vi "Photodiode-test.vi"() -> ()   [LabVIEW 2015]
uses:
  PDE_State_Machine_12_12_2016_LabVIEW_15/StateIndicator.ctl
  PDE_State_Machine_12_12_2016_LabVIEW_15/PDEState.ctl
  <vilib>/DAQmx/read.llb/DAQmx Read.vi
  <vilib>/DAQmx/read.llb/DAQmx Read (Analog 1D Wfm NChan NSamp).vi
  <vilib>/DAQmx/create/channels.llb/DAQmx Create Channel (AI-Voltage-Basic).vi
  <vilib>/DAQmx/configure/timing.llb/DAQmx Timing (Sample Clock).vi
  <vilib>/DAQmx/miscellaneous.llb/DAQmx Fill In Error Info.vi
panel:
  in  "error in":errorcluster
  out "Photodiode Values":waveform(dbl)[](graph)
  in  "Test Button":bool
  in  "Go To Idle":bool
  in  "Abort VI":bool
  out "PDE State":T1 items=["Stop VI", "Predet Fire", "Control Button", "Stop", "Connecting", "Firing", "Testing ", "Idle", "Init"]
  in  "Sample Rate (Hz)":dbl(slide)=1.0 min=0.0 max=1000000.0 step=10.0 scale=1.0..1000000.0
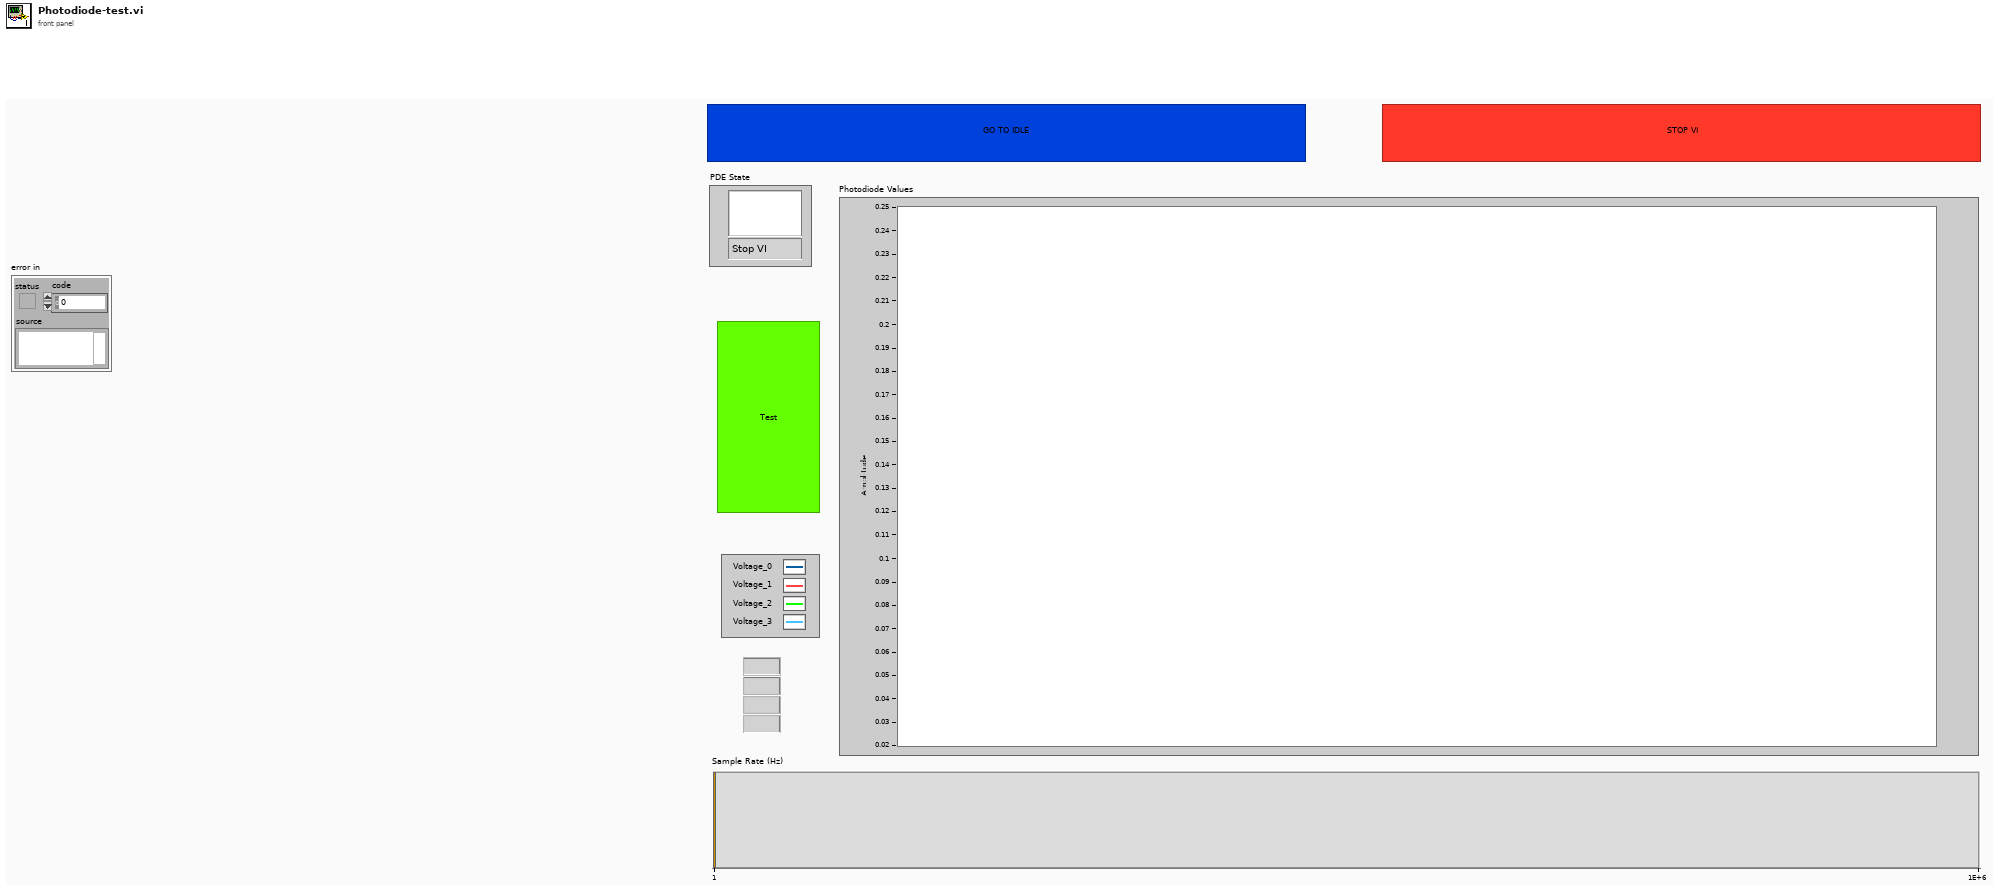
[diagram p1: front panel]
types:
  T1 = typedef "StateIndicator.ctl" = u16
  T2 = typedef "PDEState.ctl" = enum16{"Stop VI", "Predet Fire", "Control Button", "Stop", "Connecting", "Firing ", "Testing ", "Idle", "Init"}
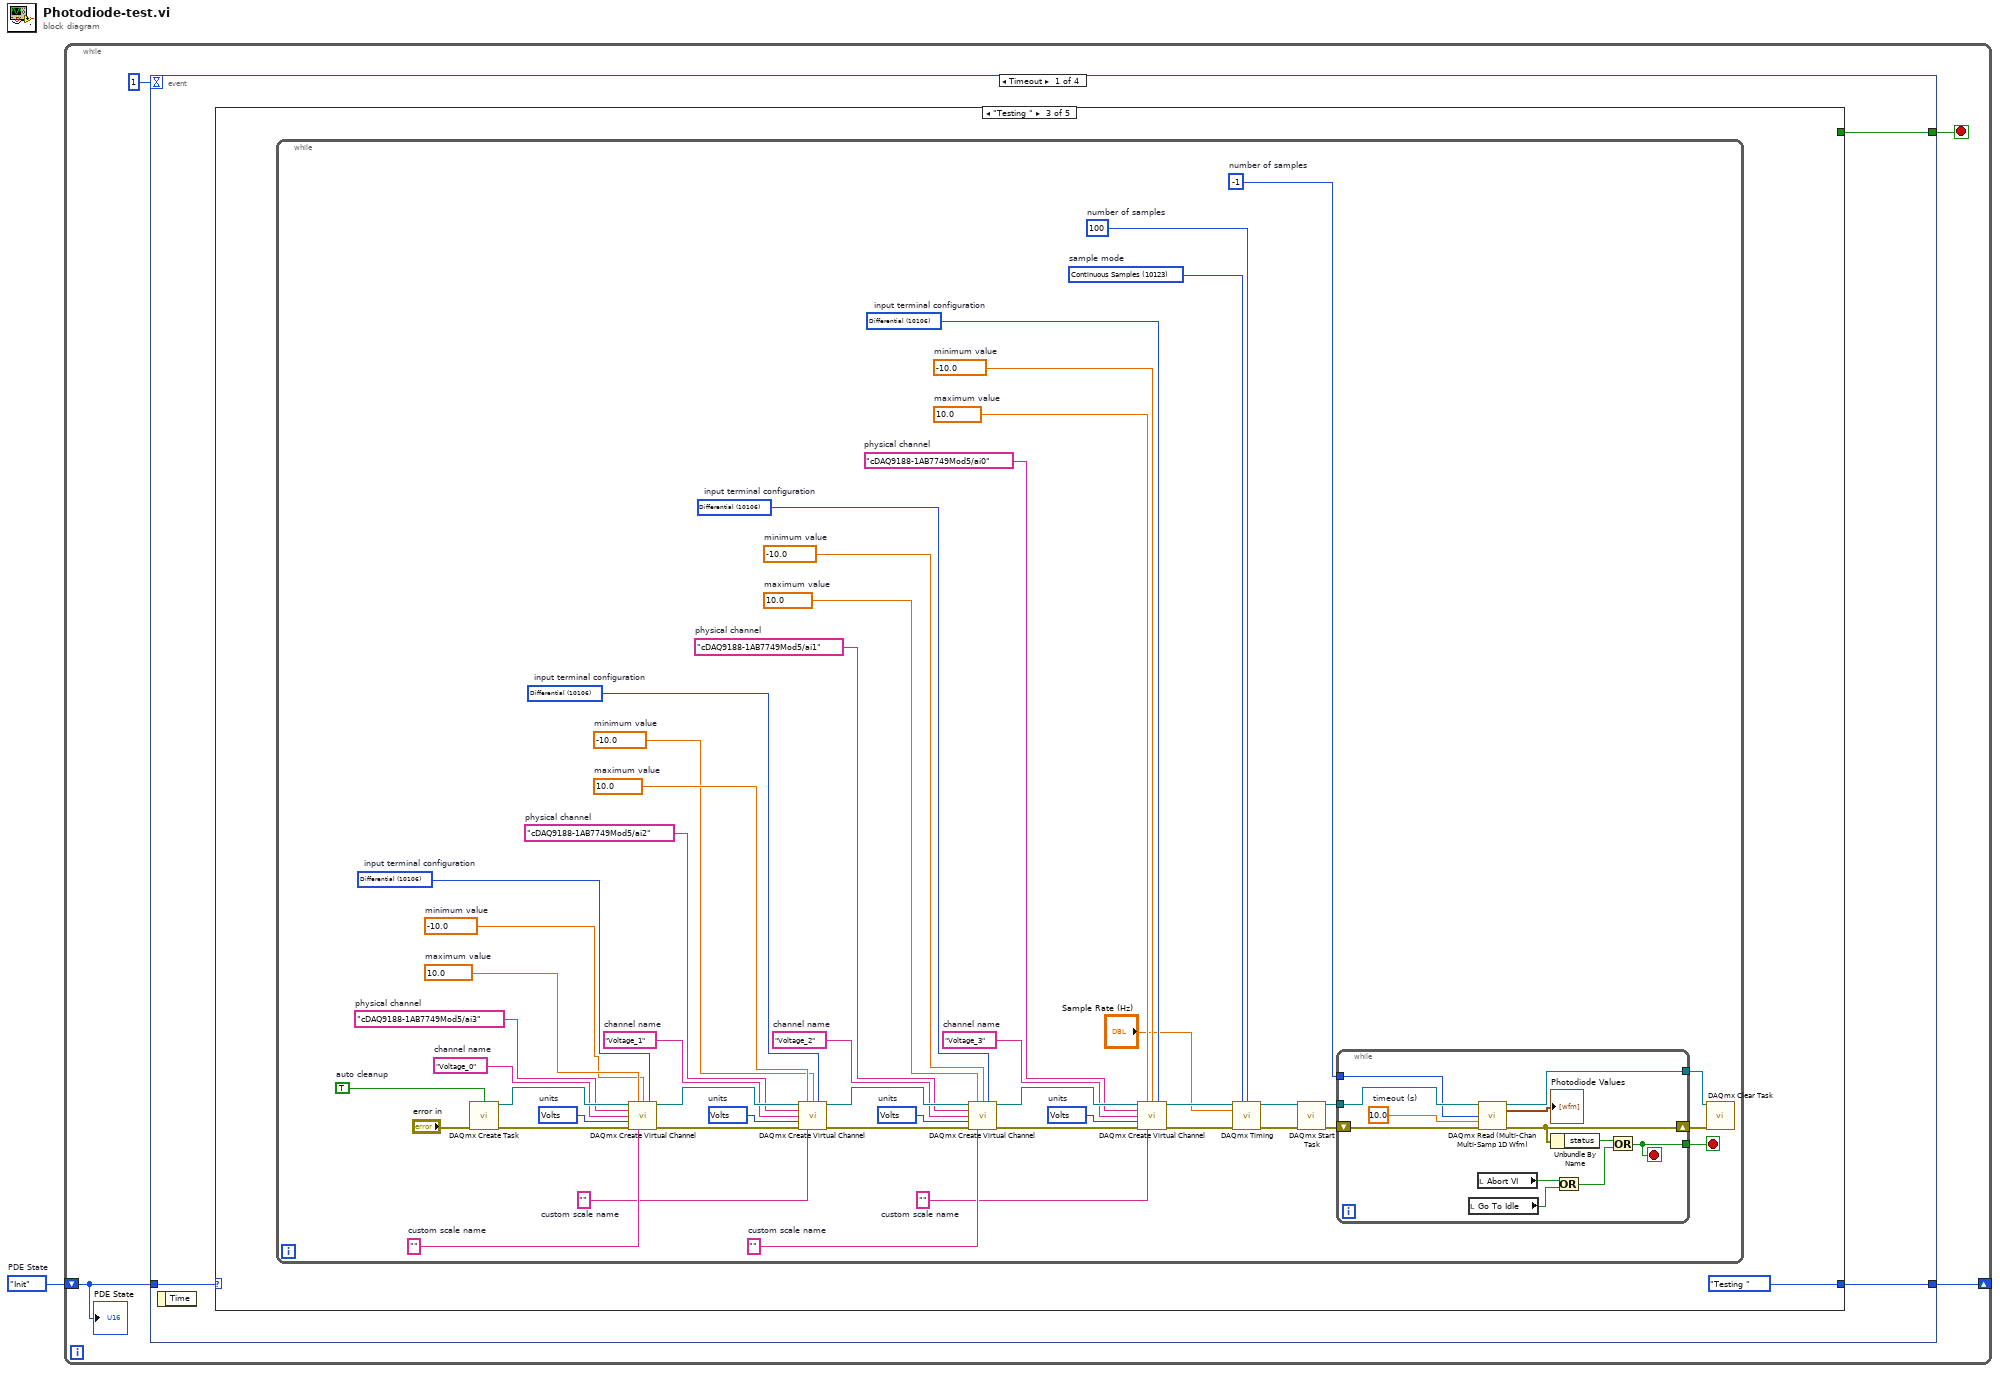
[diagram p0: block diagram]
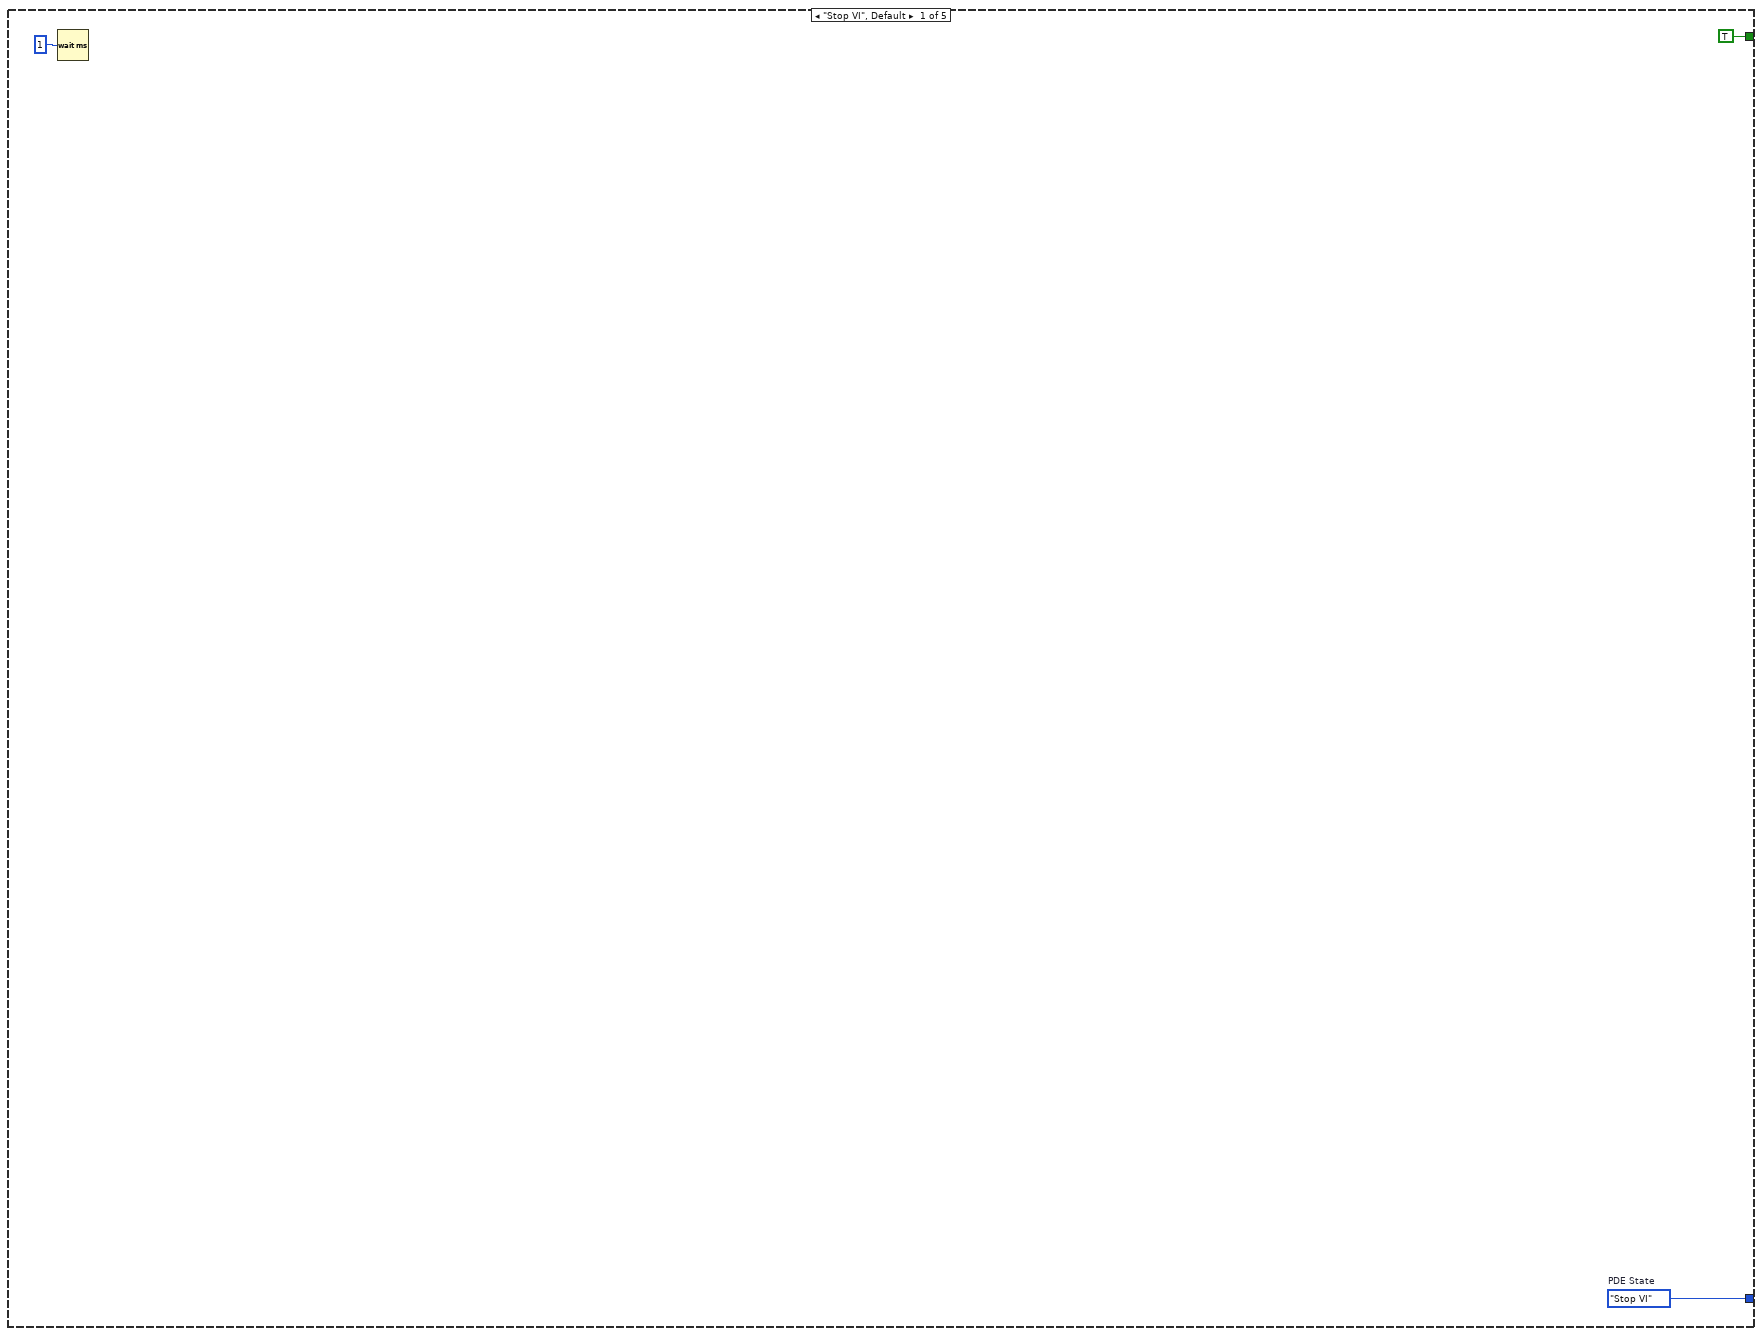
[diagram p2: hidden frame]
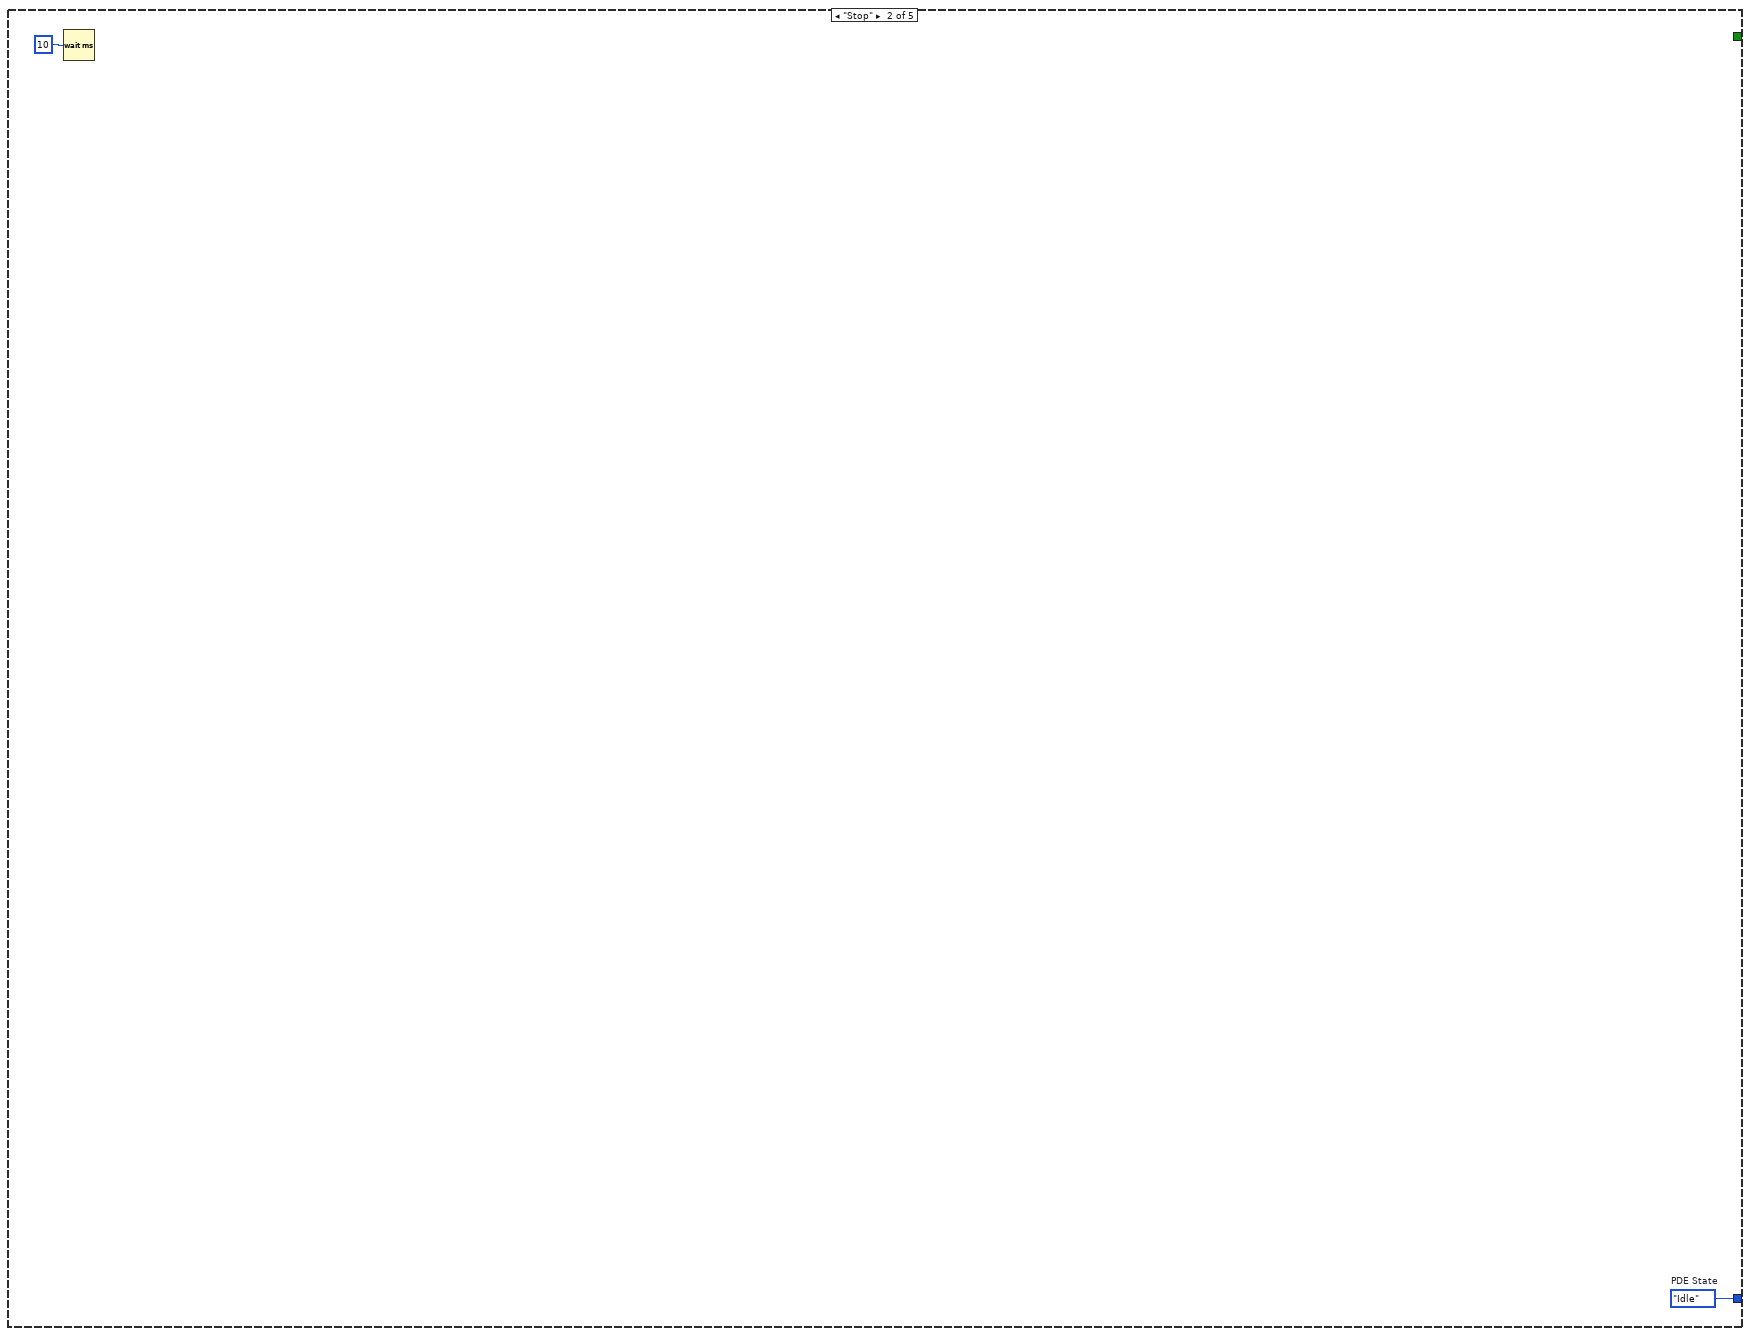
[diagram p3: hidden frame]
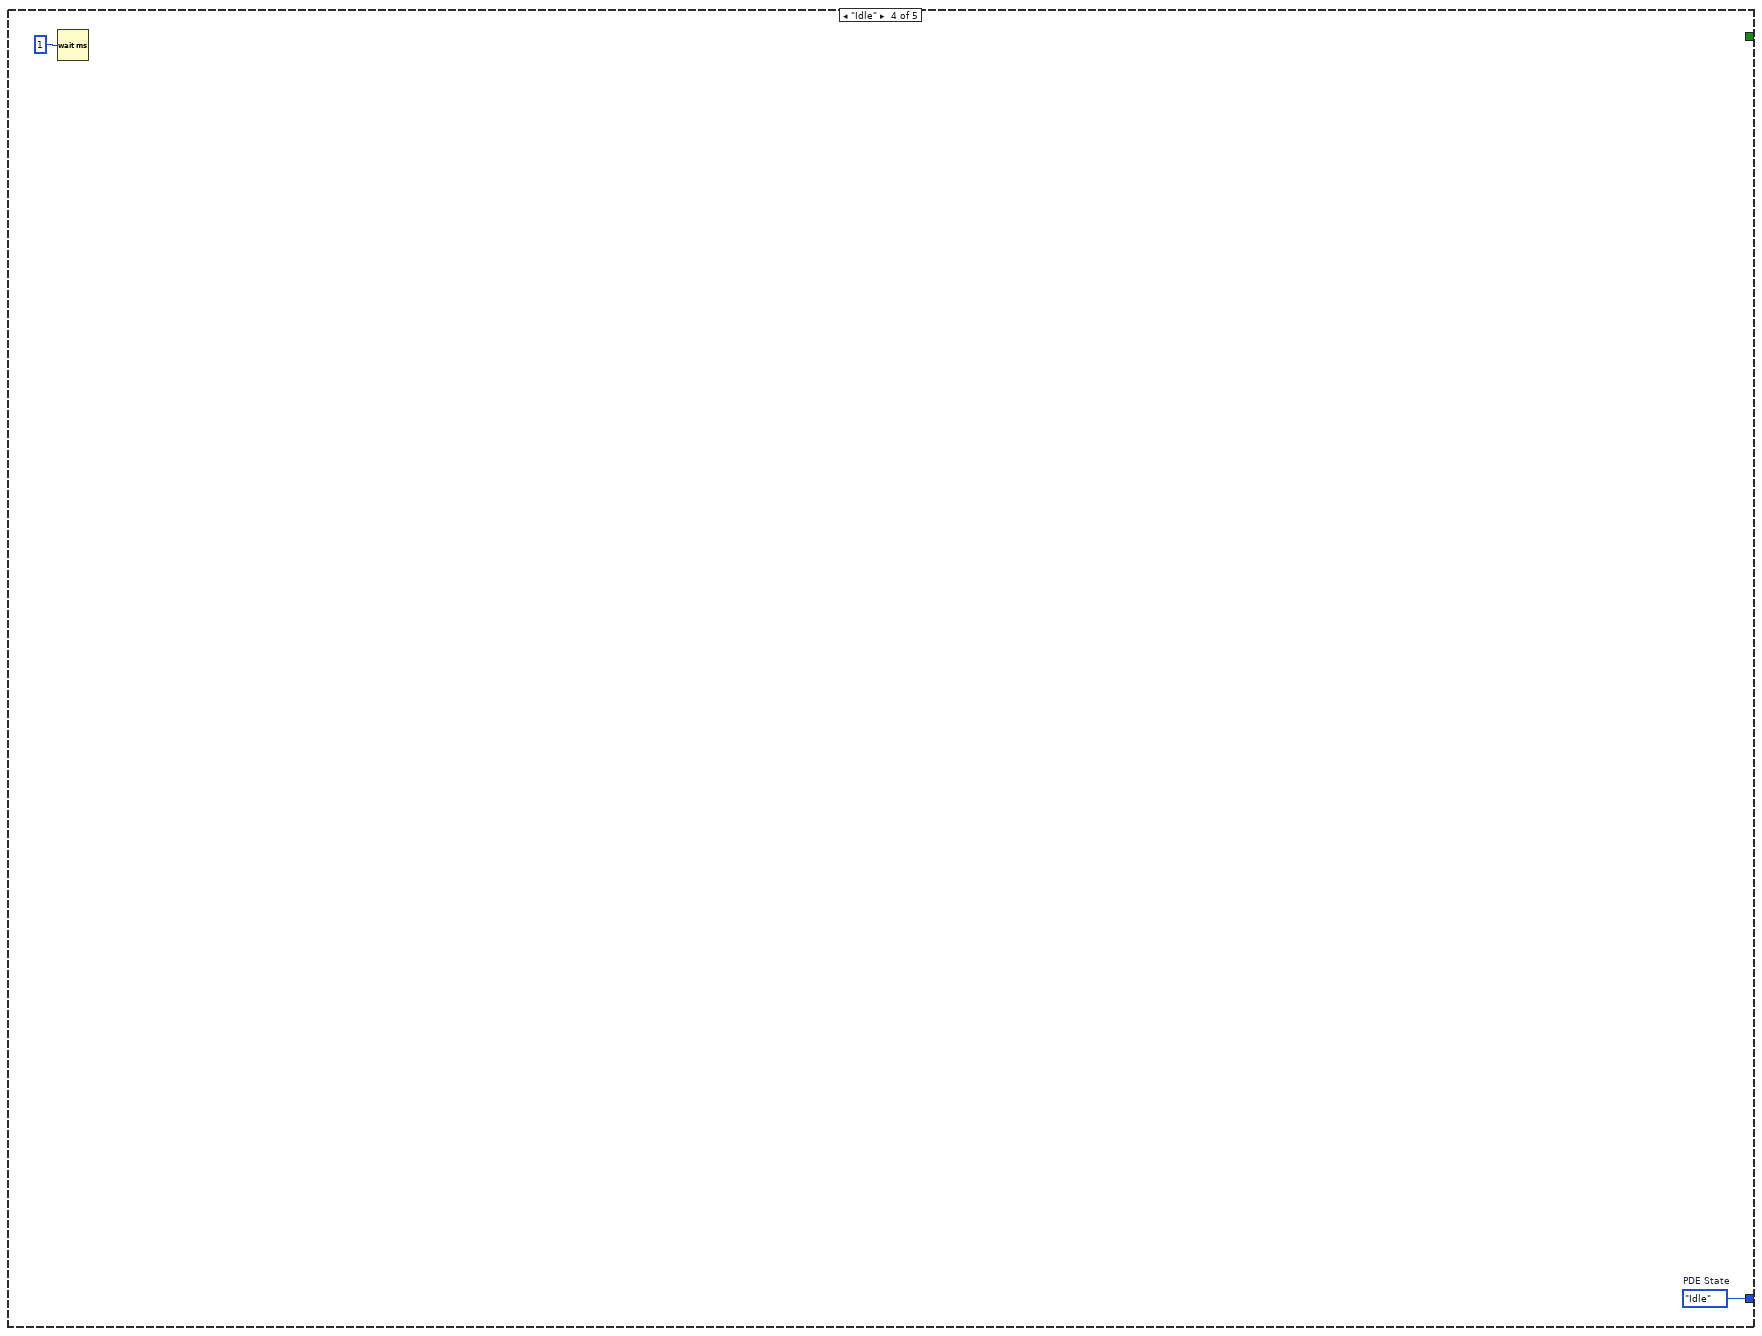
[diagram p4: hidden frame]
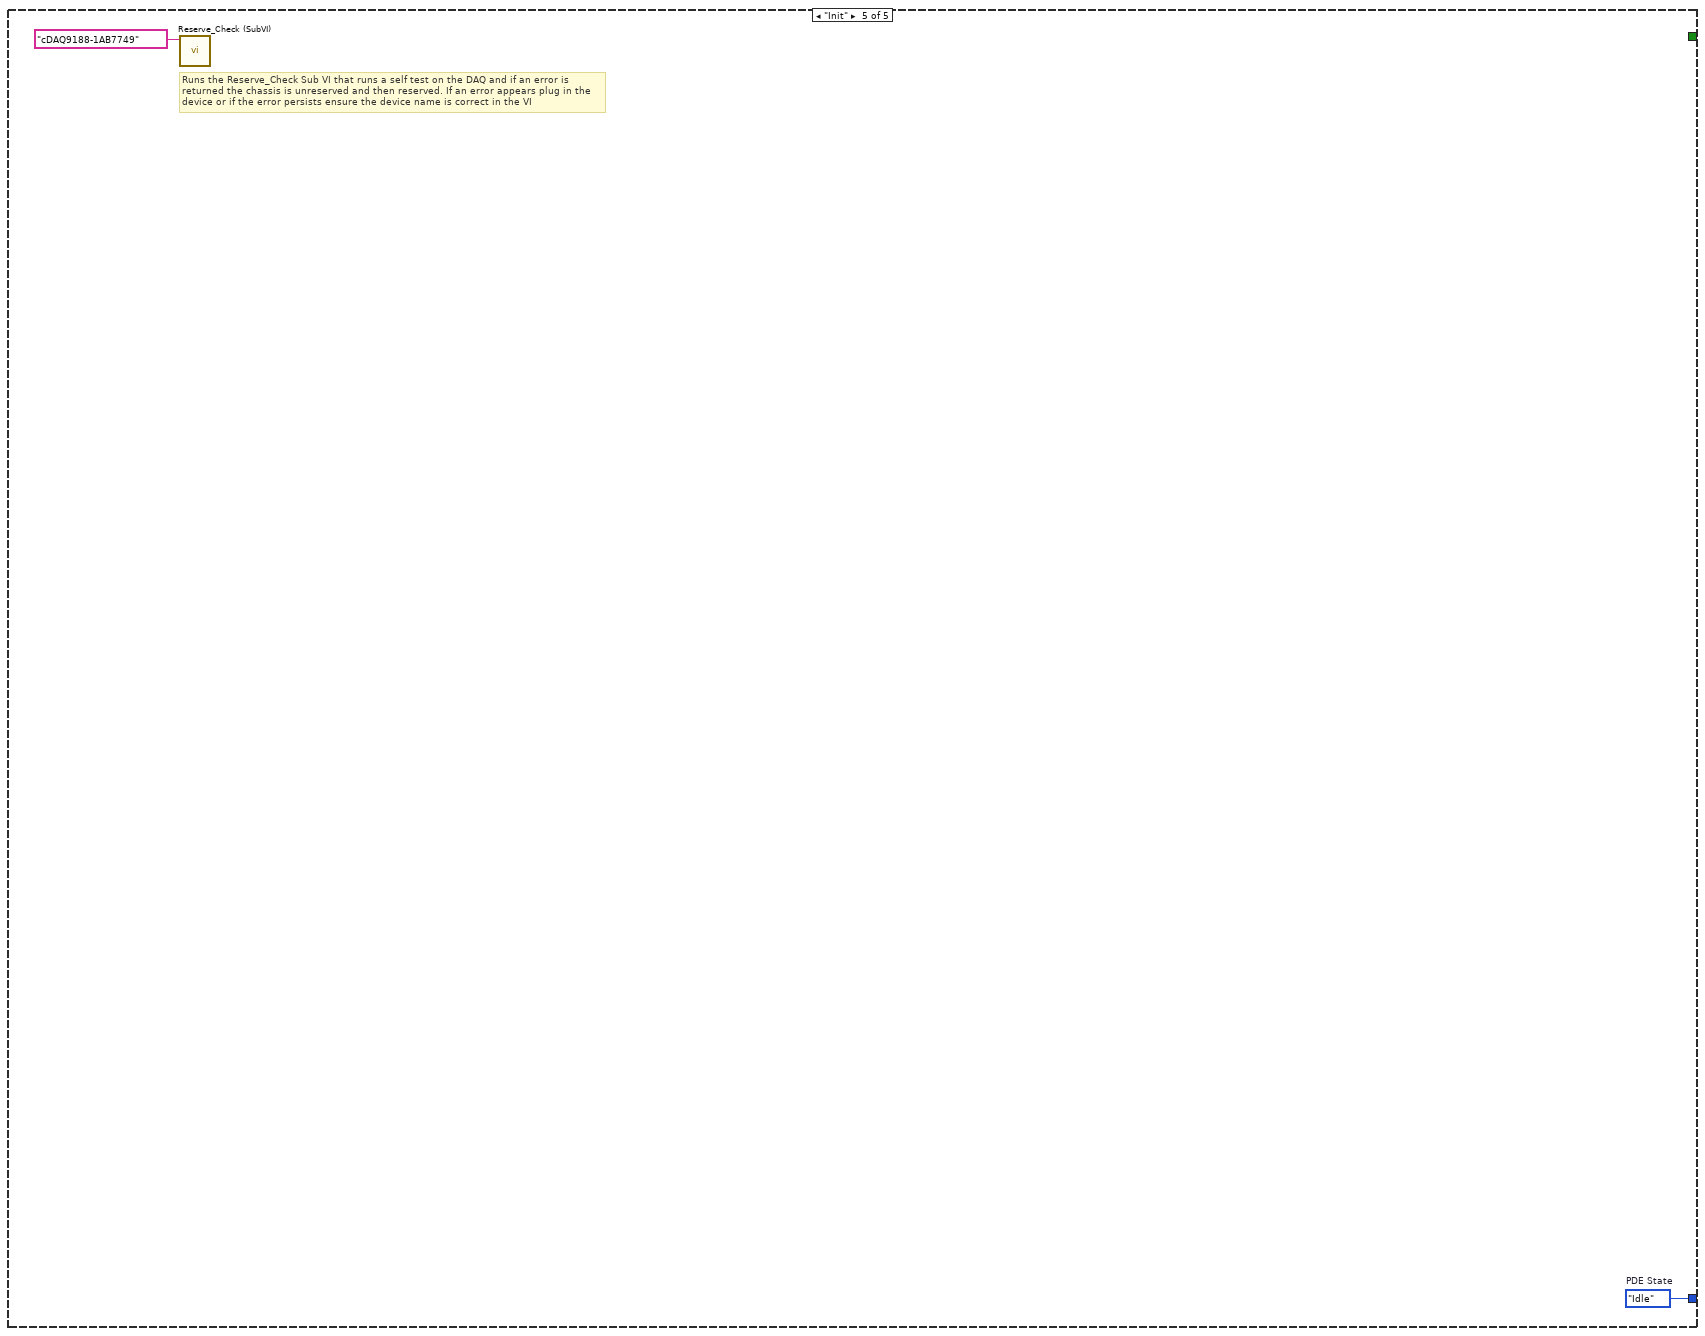
[diagram p5: hidden frame]
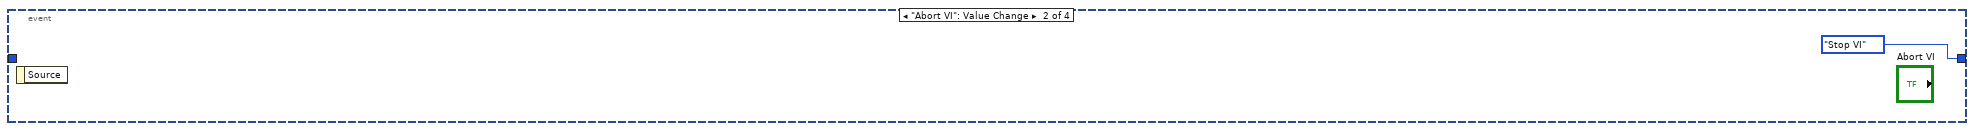
[diagram p6: hidden frame]
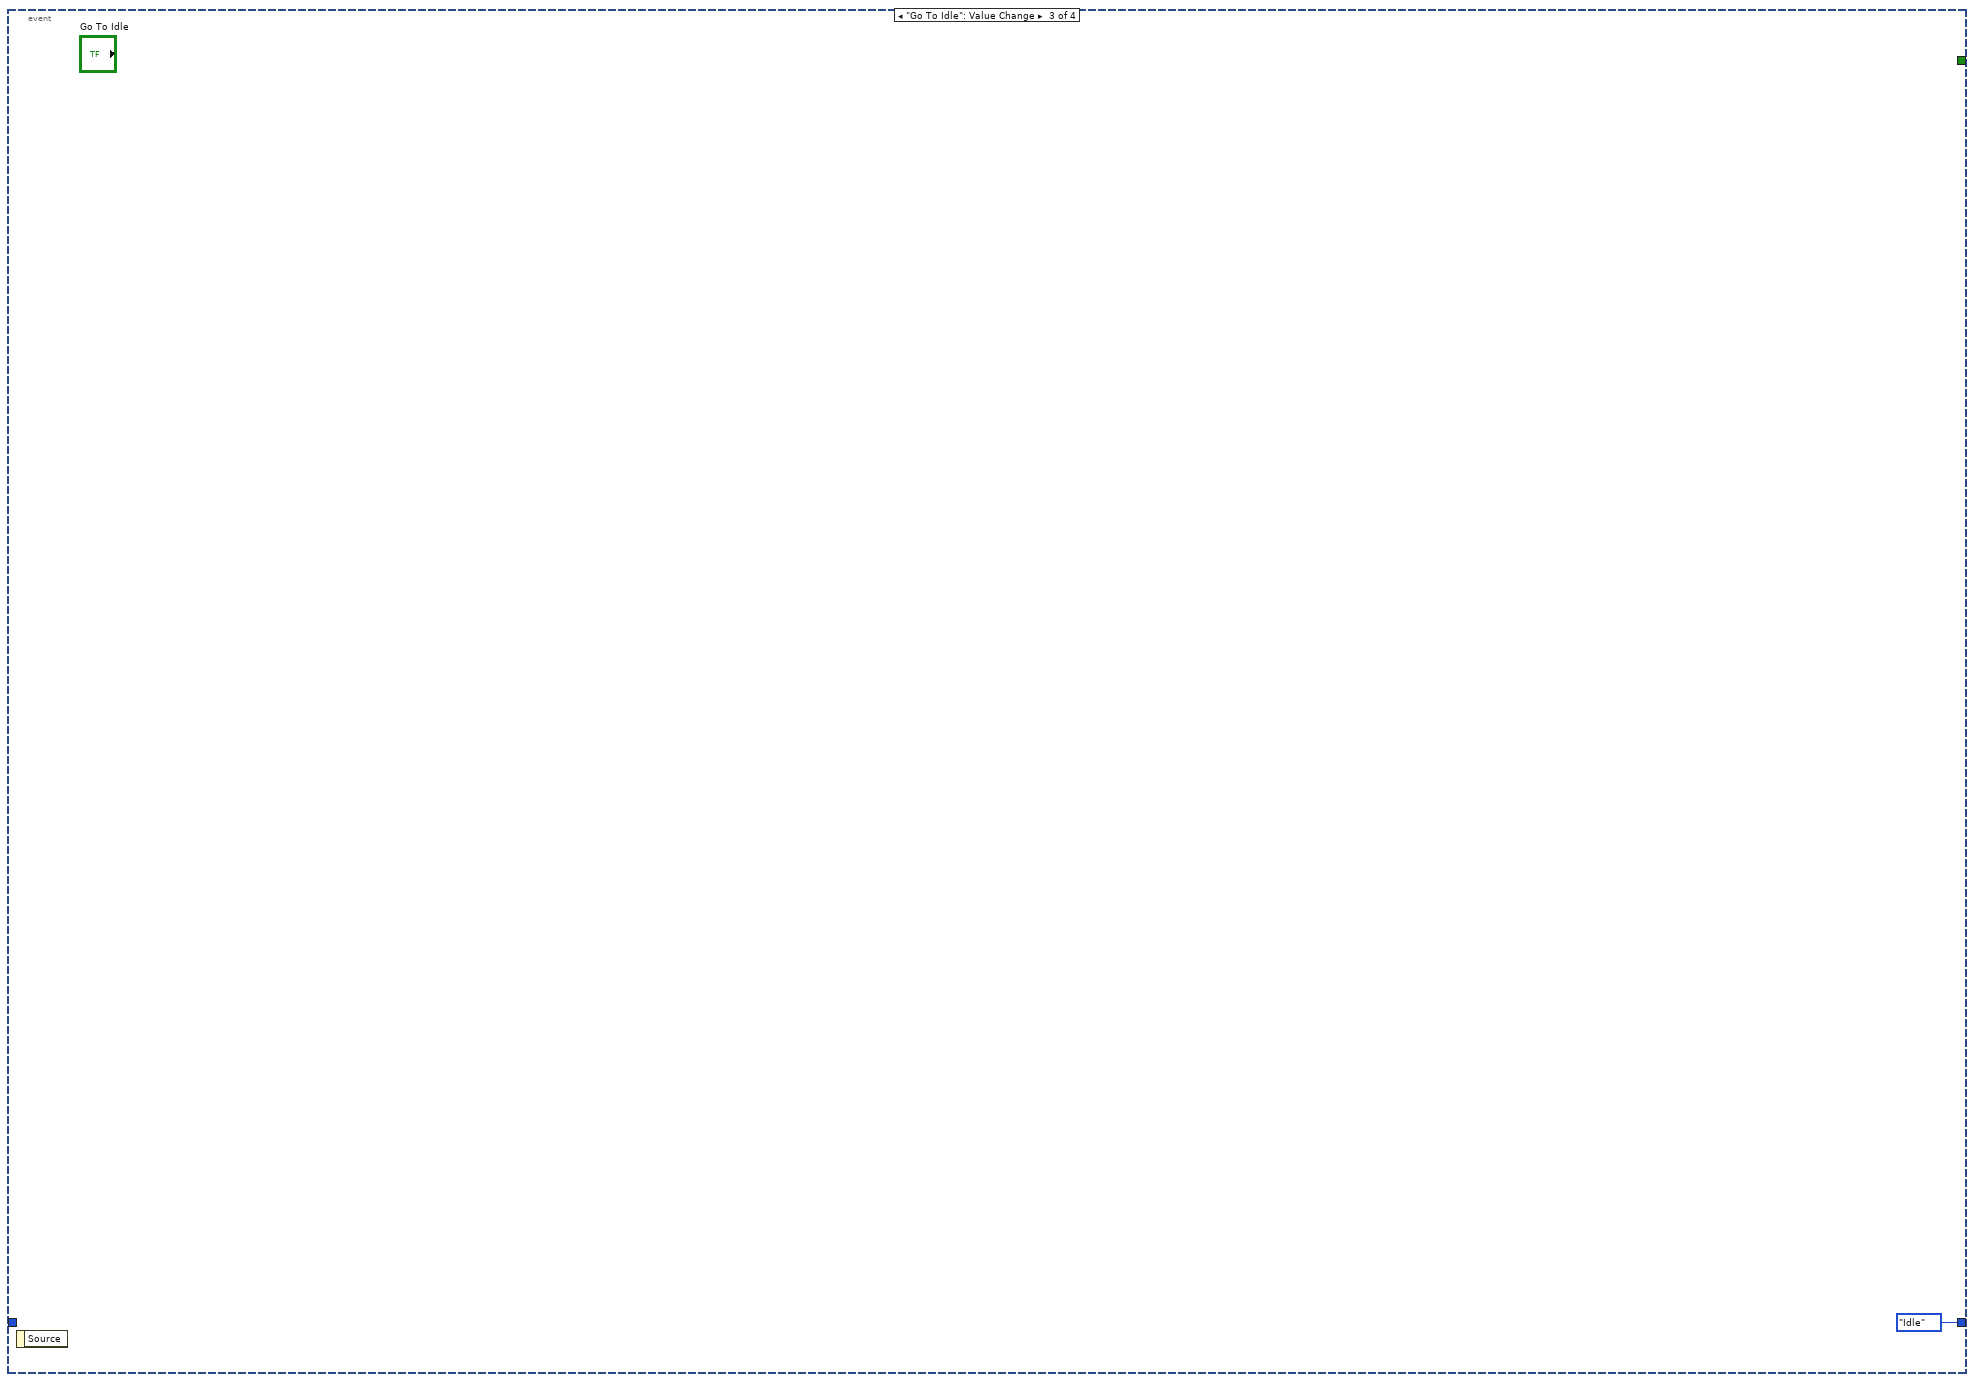
[diagram p7: hidden frame]
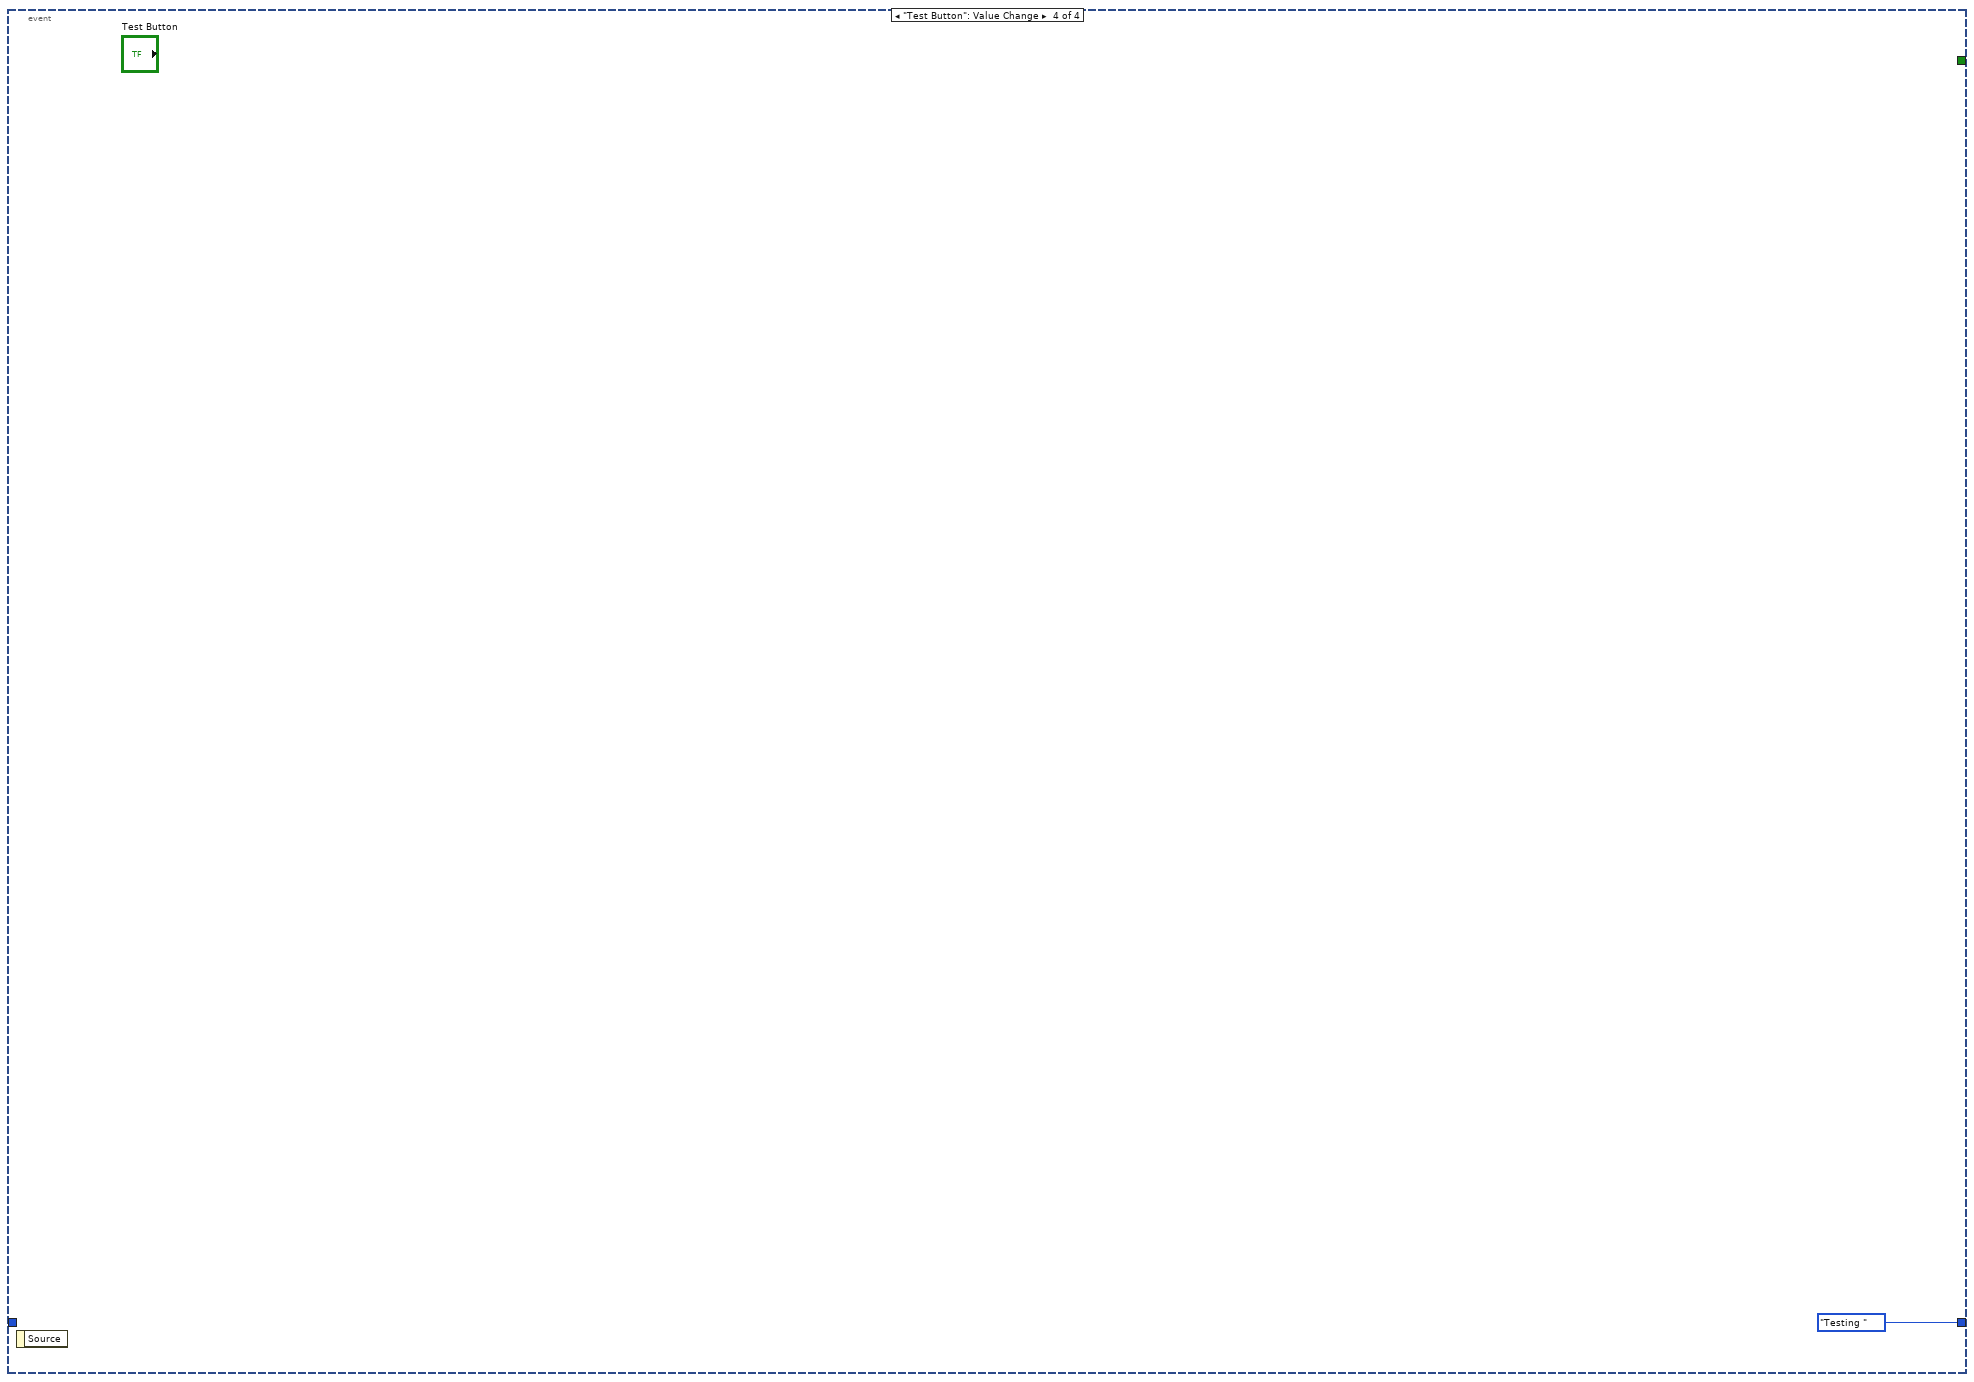
[diagram p8: hidden frame]
diagram:
  w1 = PDEState."Init"  # PDE State
  n1 = while {
    shift-right: [w4] -> _
    shift-left: w1 -> [w2]
    stop <- w3 stop-if-true
    n2 = event shown="[0] Timeout" {
      selector: _ -> [_ _ _ _]
      dyn-events: _ -> [_ _ _ _]
      timeout: 1 -> [_ _ _ _]
      tunnel: w2 -> [w8 _ _ _]
      tunnel: [w7 PDEState."Stop VI" ("PDE State") PDEState."Idle" ("PDE State") PDEState."Testing " ("PDE State")] -> w4
      tunnel: [w6 _ _ _] -> w3
      event Timeout {
        n3 = event-data() -> ()  [unwired: 1 in, 1 out]
        n4 = case shown="\"Testing \"" w8 {
          tunnel: [w11 w13 PDEState."Testing " ("PDE State") w79 w81] -> w7
          tunnel: [TRUE _ _ _ _] -> w6
          frame "Stop VI", Default {
            w11 = PDEState."Stop VI"  # PDE State
            n5 = Wait (ms)(milliseconds to wait=u32 1 ("millisecond timer value")) -> ()  [unwired: 1 out]
          }
          frame "Stop" {
            w13 = PDEState."Idle"  # PDE State
            n6 = Wait (ms)(milliseconds to wait=u32 10 ("millisecond timer value")) -> ()  [unwired: 1 out]
          }
          frame "Testing " {
            n7 = while {
              stop <- w60 stop-if-true
              w18 = 10123 items=["Finite Samples"=10178, "Continuous Samples"=10123, "Hardware Timed Single Point"=12522]  # sample mode
              w19 = 100  # number of samples
              w21 = 10106 items=["default"=-1, "RSE"=10083, "NRSE"=10078, "Differential"=10106, "Pseudodifferential"=12529]  # input terminal configuration
              w22 = 10348 items=["Volts"=10348, "From Custom Scale"=10065]  # units
              w23 = "Voltage_3"  # channel name
              w25 = ""  # custom scale name
              w26 = -10.0  # minimum value
              w27 = 10.0  # maximum value
              w28 = "cDAQ9188-1AB7749Mod5/ai0"  # physical channel
              w30 = 10106 items=["default"=-1, "RSE"=10083, "NRSE"=10078, "Differential"=10106, "Pseudodifferential"=12529]  # input terminal configuration
              w31 = 10348 items=["Volts"=10348, "From Custom Scale"=10065]  # units
              w32 = "Voltage_2"  # channel name
              w34 = ""  # custom scale name
              w35 = -10.0  # minimum value
              w36 = 10.0  # maximum value
              w37 = "cDAQ9188-1AB7749Mod5/ai1"  # physical channel
              w39 = 10106 items=["default"=-1, "RSE"=10083, "NRSE"=10078, "Differential"=10106, "Pseudodifferential"=12529]  # input terminal configuration
              w40 = 10348 items=["Volts"=10348, "From Custom Scale"=10065]  # units
              w41 = "Voltage_1"  # channel name
              w43 = ""  # custom scale name
              w44 = -10.0  # minimum value
              w45 = 10.0  # maximum value
              w46 = "cDAQ9188-1AB7749Mod5/ai2"  # physical channel
              w48 = 10106 items=["default"=-1, "RSE"=10083, "NRSE"=10078, "Differential"=10106, "Pseudodifferential"=12529]  # input terminal configuration
              w49 = 10348 items=["Volts"=10348, "From Custom Scale"=10065]  # units
              w50 = "Voltage_0"  # channel name
              w52 = ""  # custom scale name
              w53 = -10.0  # minimum value
              w54 = 10.0  # maximum value
              w55 = "cDAQ9188-1AB7749Mod5/ai3"  # physical channel
              w57 = TRUE  # auto cleanup
              w63 = -1  # number of samples
              n8 = call <vilib>:"DAQmx Create Task.vi"("auto cleanup"=w57, "error in"="error in") -> ("task out"=w56:refnum<k21>, "error out"=w58:errorcluster)  [unwired: 12 in]
              n9 = call-poly <vilib>:"DAQmx Create Virtual Channel.vi"("task in"=w56, "maximum value"=w54, "minimum value"=w53, "input terminal configuration"=w48, "physical channels"=w55, "name to assign"=w50, "units"=w49, "error in"=w58, "custom scale name"=w52) -> ("task out"=w47:refnum<k21>, "error out"=w51:errorcluster)  [unwired: 5 in]
              n10 = call-poly <vilib>:"DAQmx Create Virtual Channel.vi"("task in"=w47, "maximum value"=w45, "minimum value"=w44, "input terminal configuration"=w39, "physical channels"=w46, "name to assign"=w41, "units"=w40, "error in"=w51, "custom scale name"=w43) -> ("task out"=w38:refnum<k21>, "error out"=w42:errorcluster)  [unwired: 5 in]
              n11 = call-poly <vilib>:"DAQmx Create Virtual Channel.vi"("task in"=w38, "maximum value"=w36, "minimum value"=w35, "input terminal configuration"=w30, "physical channels"=w37, "name to assign"=w32, "units"=w31, "error in"=w42, "custom scale name"=w34) -> ("task out"=w29:refnum<k21>, "error out"=w33:errorcluster)  [unwired: 5 in]
              n12 = call-poly <vilib>:"DAQmx Create Virtual Channel.vi"("task in"=w29, "maximum value"=w27, "minimum value"=w26, "input terminal configuration"=w21, "physical channels"=w28, "name to assign"=w23, "units"=w22, "error in"=w33, "custom scale name"=w25) -> ("task out"=w20:refnum<k21>, "error out"=w24:errorcluster)  [unwired: 5 in]
              n13 = call-poly <vilib>:"DAQmx Timing.vi"("task/channels in"=w20, "sample mode"=w18, "samples per channel"=w19, "rate"="Sample Rate (Hz)", "error in"=w24) -> ("task out"=w17:refnum<k21>, "error out"=w16:errorcluster)  [unwired: 9 in]
              n14 = call <vilib>:"DAQmx Start Task.vi"("task/channels in"=w17, "error in"=w16) -> ("task out"=w65:refnum<k21>, "error out"=w64:errorcluster)  [unwired: 12 in]
              n15 = while {
                tunnel: w65 -> [w77]
                tunnel: w63 -> [w74]
                tunnel: [w75] -> w61
                shift-right: [w72] -> w62
                shift-left: w64 -> [w76]
                tunnel: [w69] -> w60
                stop <- w69 stop-if-true
                w71 = 10.0  # timeout (s)
                n16 = local read "Go To Idle"() -> (w67:bool)
                n17 = local read "Abort VI"() -> (w68:bool)
                n18 = call-poly "DAQmx Read (Multi-Chan Multi-Samp 1D Wfm).vi"("task/channels in"=w77, "number of samples per channel"=w74, "timeout"=w71, "error in"=w76) -> ("task out"=w75:refnum<k21>, "data"=→"Photodiode Values":waveform(dbl)[], "error out"=w72:errorcluster)  [unwired: 9 in]
                n19 = Unbundle By Name(w72) -> ("status"=w73:bool)
                n20 = Or(x=w68, y=w67) -> (x .or. y?=w66:bool)
                n21 = Or(x=w73, y=w66) -> (x .or. y?=w69:bool)
              }
              n22 = call <vilib>:"DAQmx Clear Task.vi"("task in"=w61, "error in"=w62) -> ()  [unwired: 13 in, 1 out]
            }
          }
          frame "Idle" {
            w79 = PDEState."Idle"  # PDE State
            n23 = Wait (ms)(milliseconds to wait=u32 1 ("millisecond timer value")) -> ()  [unwired: 1 out]
          }
          frame "Init" {
            w81 = PDEState."Idle"  # PDE State
            # "Runs the Reserve_Check Sub VI that runs a self test on the DAQ and if an error is returned the chassis is unreserved and then reserved. If an error appears plug in the device or if the error persists ensure the device name is correct in the VI"
            n24 = call "Reserve_Check (SubVI).vi"("device in"=tag "cDAQ9188-1AB7749") -> ()  [unwired: 11 in]
          }
        }
      }
      event "Abort VI": Value Change {
        n25 = event-data() -> ()  [unwired: 1 in, 1 out]
      }
      event "Go To Idle": Value Change {
        n26 = event-data() -> ()  [unwired: 1 in, 1 out]
      }
      event "Test Button": Value Change {
        n27 = event-data() -> ()  [unwired: 1 in, 1 out]
      }
    }
    "PDE State" <- w2
  }
